vi "UpdateParamsAotfArcLaser.vi"(7 "queue out":refnum<queue>) -> (1 "error out":errorcluster)   [LabVIEW 2011]
uses:
  Utilities/controls/ctlSeqFNs_Main.ctl
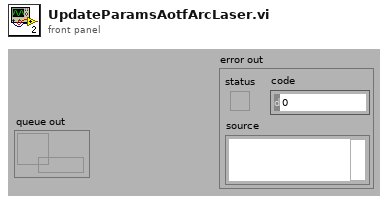
[diagram p1: front panel]
types:
  T1 = typedef "ctlSeqFNs_Main.ctl" = enum16{"ERROR", "INIT", "CONFIGURE", "MEASUREMENT", "SHUTDOWN", "IDLE", "EXIT"}
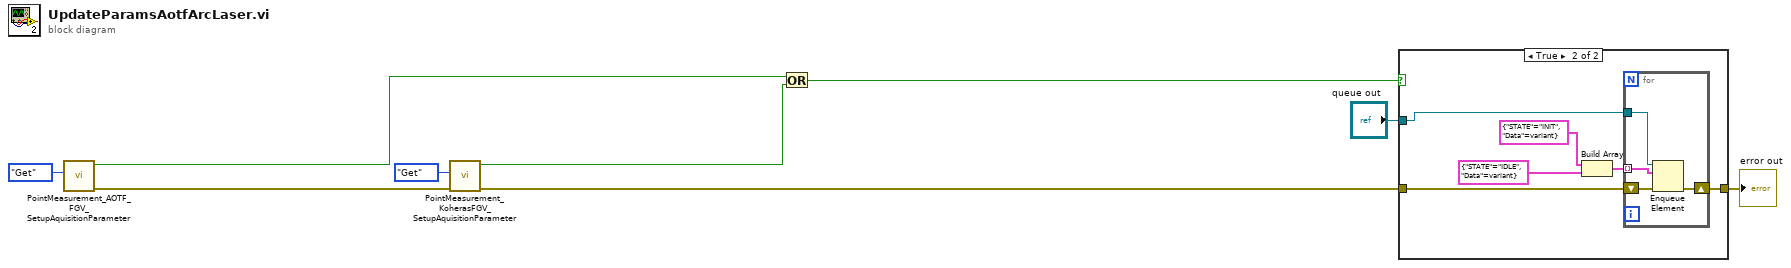
[diagram p0: block diagram]
diagram:
  n1 = call "PointMeasurement_AOTF_FGV_SetupAquisitionParameter.vi"("FGV_Control"=enum16{"Set", "Get"}."Get") -> ("error out"=w4:errorcluster, "Get"=w7:bool)  [unwired: 9 in]
  n2 = call "PointMeasurement_KoherasFGV_SetupAquisitionParameter.vi"("error in"=w4, "FGV_Control"=enum16{"Set", "Get"}."Get") -> ("error out"=w1:errorcluster, "Get"=w8:bool)  [unwired: 8 in]
  n3 = Or(x=w7, y=w8) -> (x .or. y?=w6:bool)
  n4 = case shown="True" w6 {
    tunnel: w1 -> [w10 w13]
    tunnel: [w10 w11] -> w2
    tunnel: "queue out" -> [_ w12]
    frame False {
    }
    frame True {
      n5 = Build Array(cluster{"STATE":T1, "Data":variant} {"STATE"=enum."INIT", "Data"=variant} ("element"), cluster{"STATE":T1, "Data":variant} {"STATE"=enum."IDLE", "Data"=variant} ("element")) -> (w16:cluster{"STATE":T1, "Data":variant}[])
      n6 = for {
        tunnel: w12 -> [w20]
        tunnel: w16 -> [w19] mode=indexing
        shift-right: [w18] -> w11
        shift-left: w13 -> [w17]
        n7 = Enqueue Element(queue=w20, element=w19, error in (no error)=w17) -> (error out=w18:errorcluster)  [unwired: 1 in, 2 out]
      }
    }
  }
  "error out" <- w2
